vi "set_Ga.vi"(0 "Active":bool, 1 "GAMFC3":dbl, 2 "GAMFC2":dbl, 3 "GAMFC1":dbl, 5 "Bubbler In":bool, 7 "H2 Dilute":bool, 9 "Run":bool, 11 "Remote":bool=TRUE) -> ()   [LabVIEW 2011]
uses:
  low_level_proc/globals.vi
  editor_lib/Flow_Globals.vi
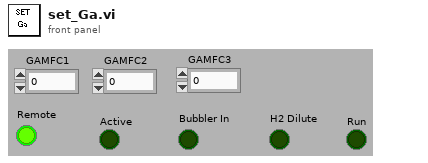
[diagram p1: front panel]
types:
  T1 = typedef "relaySpec.ctl" = cluster{"Card Index":u16, "Relay Index":u16}
  T2 = typedef "DA_Spec.ctl" = cluster{"Card Index":u16, "Channel Index":u16}
  T3 = typedef "AD_Spec.ctl" = u16
  T4 = cluster{"Relay Functions":cluster{"Remote":T1, "Active":T1, "Bubbler In":T1, "H2 dilute":T1, "Run":T1}, "D/A Functions":cluster{"Flow 1":T2, "Flow 2":T2, "Flow 3":T2}, "Flow Ranges":cluster{"Flow 1 (GAMFC1)":u16, "Flow 2 (GAMFC2)":u16, "Flow 3 (GAMFC3)":u16}, "A/D Functions":cluster{"Flow 1":T3, "Flow 2":T3, "Flow 3":T3}}
  T5 = cluster{"Remote":T1, "Active":T1, "Bubbler In":T1, "H2 dilute":T1, "Run":T1}
  T6 = cluster{"Flow 1 (GAMFC1)":u16, "Flow 2 (GAMFC2)":u16, "Flow 3 (GAMFC3)":u16}
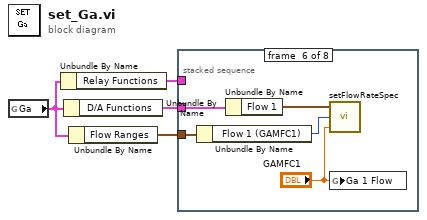
[diagram p0: block diagram]
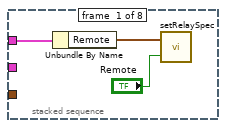
[diagram p2: hidden frame]
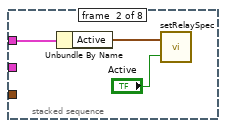
[diagram p3: hidden frame]
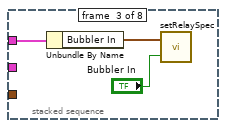
[diagram p4: hidden frame]
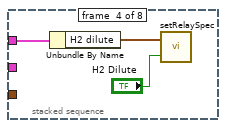
[diagram p5: hidden frame]
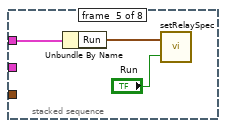
[diagram p6: hidden frame]
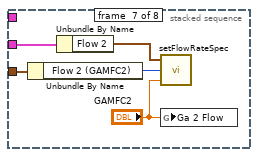
[diagram p7: hidden frame]
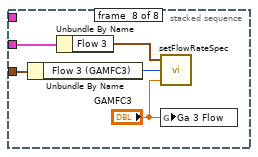
[diagram p8: hidden frame]
diagram:
  n1 = global read "globals.vi" "Ga"() -> (w2:T4)
  n2 = Unbundle By Name(w2) -> ("Relay Functions"=w4:T5)
  n3 = Unbundle By Name(w2) -> ("D/A Functions"=w3:cluster{"Flow 1":T2, "Flow 2":T2, "Flow 3":T2})
  n4 = Unbundle By Name(w2) -> ("Flow Ranges"=w1:T6)
  n5 = stacked-sequence {
    tunnel: w4 -> [w6 w9 w12 w15 w18 _ _ _]
    tunnel: w3 -> [_ _ _ _ _ w24 w28 w32]
    tunnel: w1 -> [_ _ _ _ _ w20 w26 w33]
    frame #0 {
      n6 = Unbundle By Name(w6) -> ("Remote"=w5:T1)
      n7 = call "setRelaySpec.vi"("Relay Status"="Remote", "RelaySpec"=w5) -> ()  [unwired: 1 in]
    }
    frame #1 {
      n8 = Unbundle By Name(w9) -> ("Active"=w8:T1)
      n9 = call "setRelaySpec.vi"("Relay Status"="Active", "RelaySpec"=w8) -> ()  [unwired: 1 in]
    }
    frame #2 {
      n10 = Unbundle By Name(w12) -> ("Bubbler In"=w11:T1)
      n11 = call "setRelaySpec.vi"("Relay Status"="Bubbler In", "RelaySpec"=w11) -> ()  [unwired: 1 in]
    }
    frame #3 {
      n12 = Unbundle By Name(w15) -> ("H2 dilute"=w14:T1)
      n13 = call "setRelaySpec.vi"("Relay Status"="H2 Dilute", "RelaySpec"=w14) -> ()  [unwired: 1 in]
    }
    frame #4 {
      n14 = Unbundle By Name(w18) -> ("Run"=w17:T1)
      n15 = call "setRelaySpec.vi"("Relay Status"="Run", "RelaySpec"=w17) -> ()  [unwired: 1 in]
    }
    frame #5 {
      n16 = Unbundle By Name(w20) -> ("Flow 1 (GAMFC1)"=w21:u16)
      n17 = Unbundle By Name(w24) -> ("Flow 1"=w22:T2)
      n18 = call "setFlowRateSpec.vi"("Flow Rate (sccm)"="GAMFC1", "Flow range Index"=w21, "D/A Card"=w22) -> ()  [unwired: 2 in]
      n19 = global write "Flow_Globals.vi" "Ga 1 Flow"("GAMFC1") -> ()
    }
    frame #6 {
      n20 = Unbundle By Name(w26) -> ("Flow 2 (GAMFC2)"=w25:u16)
      n21 = Unbundle By Name(w28) -> ("Flow 2"=w27:T2)
      n22 = call "setFlowRateSpec.vi"("Flow Rate (sccm)"="GAMFC2", "Flow range Index"=w25, "D/A Card"=w27) -> ()  [unwired: 2 in]
      n23 = global write "Flow_Globals.vi" "Ga 2 Flow"("GAMFC2") -> ()
    }
    frame #7 {
      n24 = Unbundle By Name(w33) -> ("Flow 3 (GAMFC3)"=w30:u16)
      n25 = Unbundle By Name(w32) -> ("Flow 3"=w31:T2)
      n26 = call "setFlowRateSpec.vi"("Flow Rate (sccm)"="GAMFC3", "Flow range Index"=w30, "D/A Card"=w31) -> ()  [unwired: 2 in]
      n27 = global write "Flow_Globals.vi" "Ga 3 Flow"("GAMFC3") -> ()
    }
  }
